vi "Find max power voltage from log file.vi"(7 "Cell details cluster in 2":T1={"Measure?"=TRUE, "Area (cm^2)"=0.0, "Cell Label"="", "Cell Description"="", "Cell Position"=0, "Time in rig (s)"=0.0, "Time to next scan (s)"=0.0, "Scan number"=0.0, "When did you stick it in?"=0.0, "Time between scans (s)"=0.0, "Time of the last scan (s)"=0.0, "Scan settings in queue"=0, "Sample Holder"=0.0, "User Name"=""} {"Scan settings in queue" items=["Regular", "Inverted", "MartinaSettings"]; "Time of the last scan (s)" format="%<%H:%M:%S>t"; "When did you stick it in?" format="%<%H:%M:%S>t"; "Time to next scan (s)" format="%<%H:%M:%S>t"; "Time in rig (s)" format="%<%H:%M:%S>t"}, 9 "Pixel":i32, 11 "File path of master log":path) -> (3 "Vmp":dbl)   [LabVIEW 2011]
uses:
  Typedefs/Queue cluster.ctl
  <vilib>/Utility/file.llb/Read From Spreadsheet File (string).vi
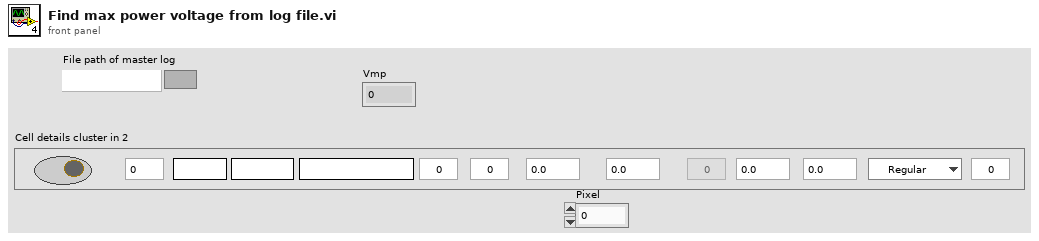
[diagram p1: front panel]
types:
  T1 = typedef "Queue cluster.ctl" = cluster{"Measure?":bool, "Area (cm^2)":dbl, "Cell Label":string, "Cell Description":string, "Cell Position":i32, "Time in rig (s)":dbl, "Time to next scan (s)":dbl, "Scan number":dbl, "When did you stick it in?":dbl, "Time between scans (s)":dbl, "Time of the last scan (s)":dbl, "Scan settings in queue":u16, "Sample Holder":dbl, "User Name":string}
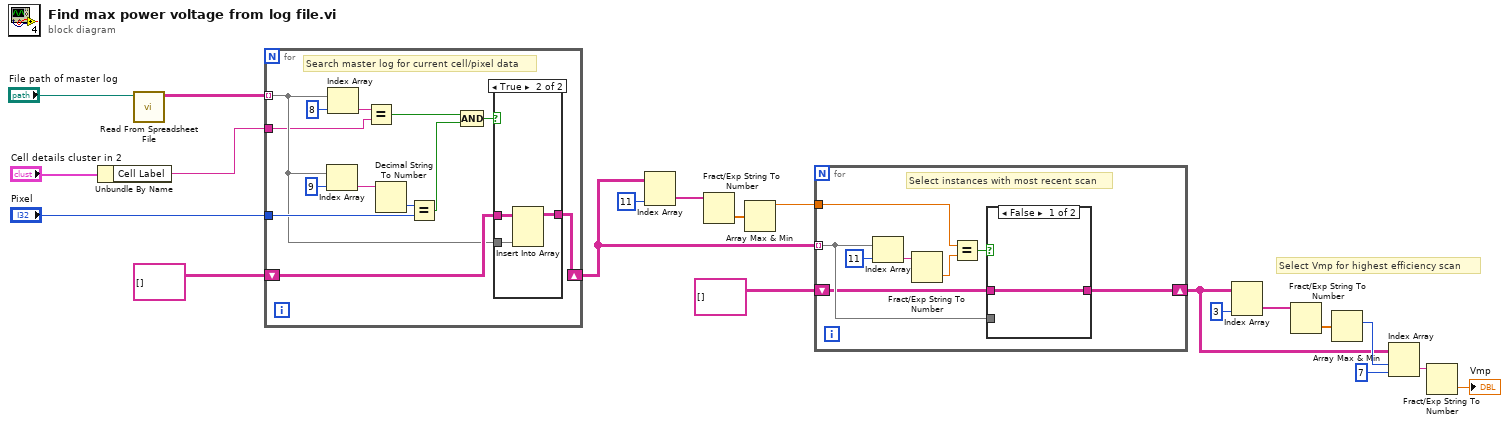
[diagram p0: block diagram]
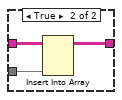
[diagram p2: hidden frame]
diagram:
  # "Select Vmp for highest efficiency scan"
  n1 = Unbundle By Name("Cell details cluster in 2") -> ("Cell Label"=w11:string)
  n2 = call-poly <vilib>:"Read From Spreadsheet File.vi"("file path (dialog if empty)"="File path of master log") -> ("all rows"=w19:string[][])  [unwired: 6 in, 4 out]
  n3 = for {
    tunnel: w19 -> [w25] mode=indexing
    shift-right: [w32] -> w8
    shift-left: string[][] [] ("all rows") -> [w33]
    tunnel: "Pixel" -> [w26]
    tunnel: w11 -> [w21]
    # "Search master log for current cell/pixel data"
    n4 = Index Array(array=w25, index=9) -> (element=w30:string)
    n5 = Index Array(array=w25, index=8) -> (element=w23:string)
    n6 = Equal?(x=w23, y=w21) -> (x = y?=w22:bool)
    n7 = Decimal String To Number(string=w30) -> (number=w29:i32)  [unwired: 2 in, 1 out]
    n8 = Equal?(x=w29, y=w26) -> (x = y?=w27:bool)
    n9 = Compound Arithmetic op=AND(w22, w27) -> (w28:bool)
    n10 = case shown="True" w28 {
      tunnel: w33 -> [w34 w37]
      tunnel: [w34 w36] -> w32
      tunnel: w25 -> [_ w35]
      frame False {
      }
      frame True {
        n11 = Insert Into Array(array=w37, new element=w35) -> (w36:string[][])  [unwired: 2 in]
      }
    }
  }
  n12 = Index Array(array=w8, index (col)=11 ("disabled index (col)")) -> (element=w10:string[])  [unwired: 1 in]
  n13 = Fract/Exp String To Number(string=w10) -> (number=w9:dbl[])  [unwired: 3 in, 1 out]
  n14 = Array Max & Min(array=w9) -> (max value=w7:dbl)  [unwired: 3 out]
  n15 = for {
    tunnel: w8 -> [w40] mode=indexing
    tunnel: w7 -> [w42]
    shift-right: [w38] -> w1
    shift-left: string[][] [] ("all rows") -> [w39]
    # "Select instances with most recent scan"
    n16 = Index Array(array=w40, index=11) -> (element=w44:string)
    n17 = Fract/Exp String To Number(string=w44) -> (number=w43:dbl)  [unwired: 3 in, 1 out]
    n18 = Equal?(x=w42, y=w43) -> (x = y?=w41:bool)
    n19 = case shown="False" w41 {
      tunnel: w40 -> [_ w49]
      tunnel: w39 -> [w46 w48]
      tunnel: [w46 w47] -> w38
      frame False {
      }
      frame True {
        n20 = Insert Into Array(array=w48, new element=w49) -> (w47:string[][])  [unwired: 2 in]
      }
    }
  }
  n21 = Index Array(array=w1, index (col)=3 ("disabled index (col)")) -> (element=w4:string[])  [unwired: 1 in]
  n22 = Fract/Exp String To Number(string=w4) -> (number=w3:dbl[])  [unwired: 3 in, 1 out]
  n23 = Array Max & Min(array=w3) -> (max index (indices)=w2:i32)  [unwired: 3 out]
  n24 = Index Array(array=w1, index (row)=w2, index (col)=7 ("disabled index (col)")) -> (element=w15:string)
  n25 = Fract/Exp String To Number(string=w15) -> (number=→"Vmp":dbl)  [unwired: 3 in, 1 out]
